vi "reset buttons.vi"(4 "error IO":errorcluster, 5 "input main cluster":T1) -> (0 "error out":errorcluster, 1 "output main cluster":T1)   [LabVIEW 2010]
uses:
  Main_cluster.ctl
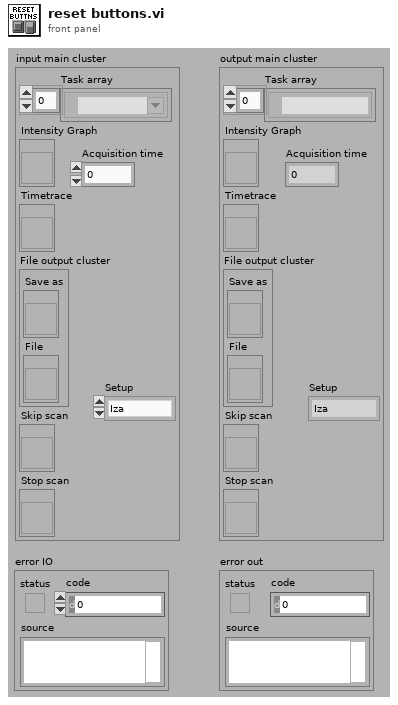
[diagram p1: front panel]
types:
  T1 = typedef "Main_cluster.ctl" = cluster{"Task array":refnum<k21>[], "Intensity Graph":refnum<vi>, "Timetrace":refnum<vi>, "File output cluster":cluster{"Save as":refnum<vi>, "File":refnum<vi>}, "Skip scan":refnum<vi>, "Stop scan":refnum<vi>, "Acquisition time":dbl, "Setup":enum16{"Iza", "Lukasz"}}
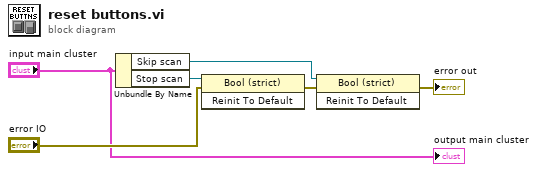
[diagram p0: block diagram]
diagram:
  n1 = Unbundle By Name("input main cluster") -> ("Skip scan"=w1:refnum<vi>, "Stop scan"=w2:refnum<vi>)
  n2 = invoke on="Invoke Node" class="Bool (strict)" method="Reinit To Default"(reference=w2, error in="error IO") -> (error out=w4:errorcluster)  [unwired: 1 in, 2 out]
  n3 = invoke on="Invoke Node" class="Bool (strict)" method="Reinit To Default"(reference=w1, error in=w4) -> (error out=→"error out":errorcluster)  [unwired: 1 in, 2 out]
  "output main cluster" <- "input main cluster"
